vi "Connect.vi"(8 "error in (no error)":errorcluster, 11 "Laser Diode Controller in":refnum<class "KLD101.lvclass">) -> (0 "error out":errorcluster, 3 "Laser Diode Controller out":refnum<class "KLD101.lvclass">)   [LabVIEW 2016, in "Laser Diode Controller.lvlib" / "KLD101.lvclass"]
uses:
  KLD101.lvclass
  KLD101.lvclass/KLD101.ctl
  TypeDefs/KLD-LaserErrors.ctl
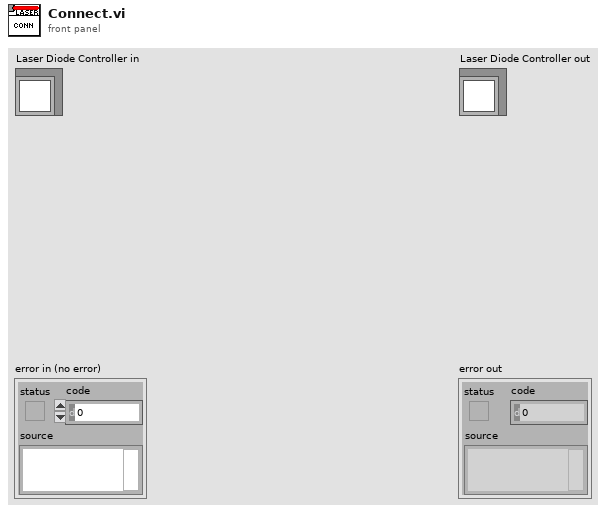
[diagram p1: front panel]
types:
  T1 = typedef "Laser Diode Controller.lvlib/KLD101.lvclass/KLD-LaserErrors.ctl" = enum16{"deviceSerialNotFound"}
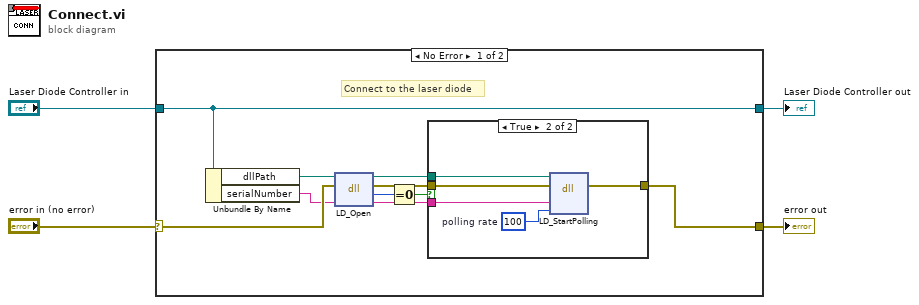
[diagram p0: block diagram]
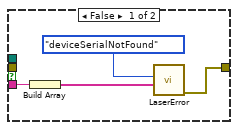
[diagram p2: hidden frame]
diagram:
  n1 = case shown="No Error" "error in (no error)" {
    selector: "error in (no error)" -> [w14 w25]
    tunnel: [w11 w25] -> w3
    tunnel: [w13 w24] -> w1
    tunnel: "Laser Diode Controller in" -> [w13 w24]
    frame No Error {
      # "Connect to the laser diode"
      n2 = Unbundle By Name(w13) -> ("dllPath"=w8:path, "serialNumber"=w6:string)
      n3 = dll-call lib="C:/IDEXX Software/Collimation/data/Thorlabs.MotionControl.KCube.LaserDiode.dll" fn="LD_Open"(path in=w8, error in=w14, "SerialNumber"=w6) -> (path out=w7:path, error out=w12:errorcluster, "return type"=w10:i32, "SerialNumber"=w5:string)  [unwired: 1 in]
      n4 = Equal To 0?(x=w10) -> (x = 0?=w9:bool)
      n5 = case shown="True" w9 {
        tunnel: w12 -> [_ w23]
        tunnel: [w15 w22] -> w11
        tunnel: w5 -> [w16 w21]
        tunnel: w7 -> [_ w19]
        frame False {
          n6 = Build Array(w16) -> (w18:string[])
          n7 = call "LaserError.vi"("args"=w18, "laserErrorType"=KLD-LaserErrors."deviceSerialNotFound") -> ("error out"=w15:errorcluster)  [unwired: 9 in]
        }
        frame True {
          w20 = i8 100  # polling rate
          n8 = dll-call lib="C:/IDEXX Software/Collimation/data/Thorlabs.MotionControl.KCube.LaserDiode.dll" fn="LD_StartPolling"(path in=w19, error in=w23, "serialNumber"=w21, "milliseconds"=w20) -> (error out=w22:errorcluster)  [unwired: 4 in, 1 out]
        }
      }
    }
    frame Error {
    }
  }
  "error out" <- w3
  "Laser Diode Controller out" <- w1
